vi "Go to Init.vi"(8 "error in (no error)":errorcluster, 11 "Init in":refnum<class "Init.lvclass">) -> (0 "error out":errorcluster, 3 "Chef State out":refnum<class "State Actor.lvclass">)   [LabVIEW 2024, in "Chef State.lvlib" / "Init.lvclass"]
uses:
  Init.lvclass
  C:/Program Files/National Instruments/LabVIEW 2024/vi.lib/NI/Actors/State Actor/State Actor/State Actor.lvclass
  <vilib>/NI/Actors/State Actor/State Actor/State Actor.lvclass
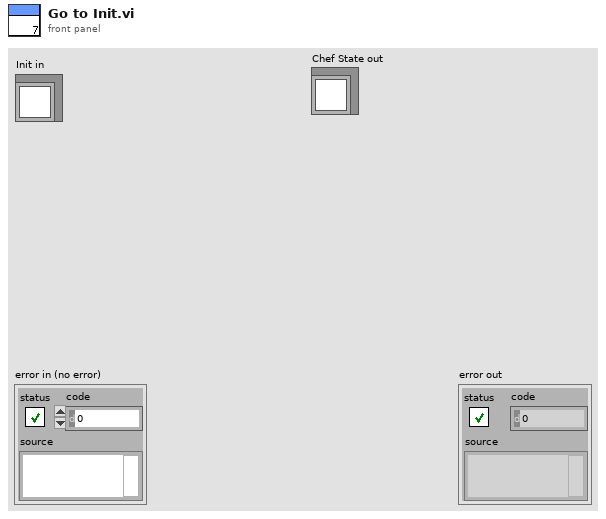
[diagram p1: front panel]
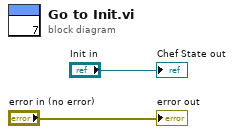
[diagram p0: block diagram]
diagram:
  "error out" <- "error in (no error)"
  "Chef State out" <- "Init in"
